vi "TS-60.vi"() -> ()   [LabVIEW 2013]
panel:
  in  "Slide 2":dbl(slide) scale=0.0..10.0
  out "ABC Ind3":bool
  out "ACB Ind 3":bool
  in  "ABC-ACB 3":bool=TRUE
  in  "Slide":dbl(slide) scale=0.0..10.0
  out "ABC Ind 2":bool
  out "ACB Ind 2":bool
  in  "ABC-ACB 2":bool=TRUE
  out "28VDC Ind":bool
  in  "28VDC":bool
  out "SPEED - FPM":dbl format="%3.1f"
  out "DOWNFORCE":dbl format="%1.1f"
  out "TRACTIVE LOAD":dbl format="%1.1f"
  in  "Stop Button":bool
  out "400Hz Ind":bool
  in  "400Hz":bool
  out "ABC Ind":bool
  out "ACB Ind":bool
  in  "ABC-ACB":bool=TRUE
  out "DC AMPS":dbl format="%.3f"
  out "DC VOLTS":dbl format="%-2.1f"
  out "AC FREQUENCY":dbl format="%4.1f"
  out "AC AMPS L3":dbl format="%1.2f"
  out "AC VOLTS L3":dbl format="%3.1f"
  out "AC AMPS L2":dbl format="%1.2f"
  out "AC VOLTS L2":dbl format="%1.1f"
  out "AC AMPS L1":dbl format="%1.2f"
  out "AC VOLTS L1":dbl format="%1.1f"
  in  "DC V":dbl(slide) scale=0.0..30.0
  in  "DC A":dbl(slide) scale=0.0..5.0
  in  "AC FREQ":dbl(slide) scale=0.0..400.0
  in  "AC VOLTS":dbl(slide) scale=0.0..115.0
  in  "AC AMPS":dbl(slide) scale=0.0..25.0
  # "SYSTEM CONTROL"
  # "28VDC"
  # "OFF"
  # "LOAD CONDITION"
  # "DOWNFORCE"
  # "UP"
  # "DOWN"
  # "TRACTION"
  # "ON"
  # "OFF"
  # "400Hz"
  # "OFF"
  # "ABC"
  # "ACB"
  # "POWER CONSUMPTION"
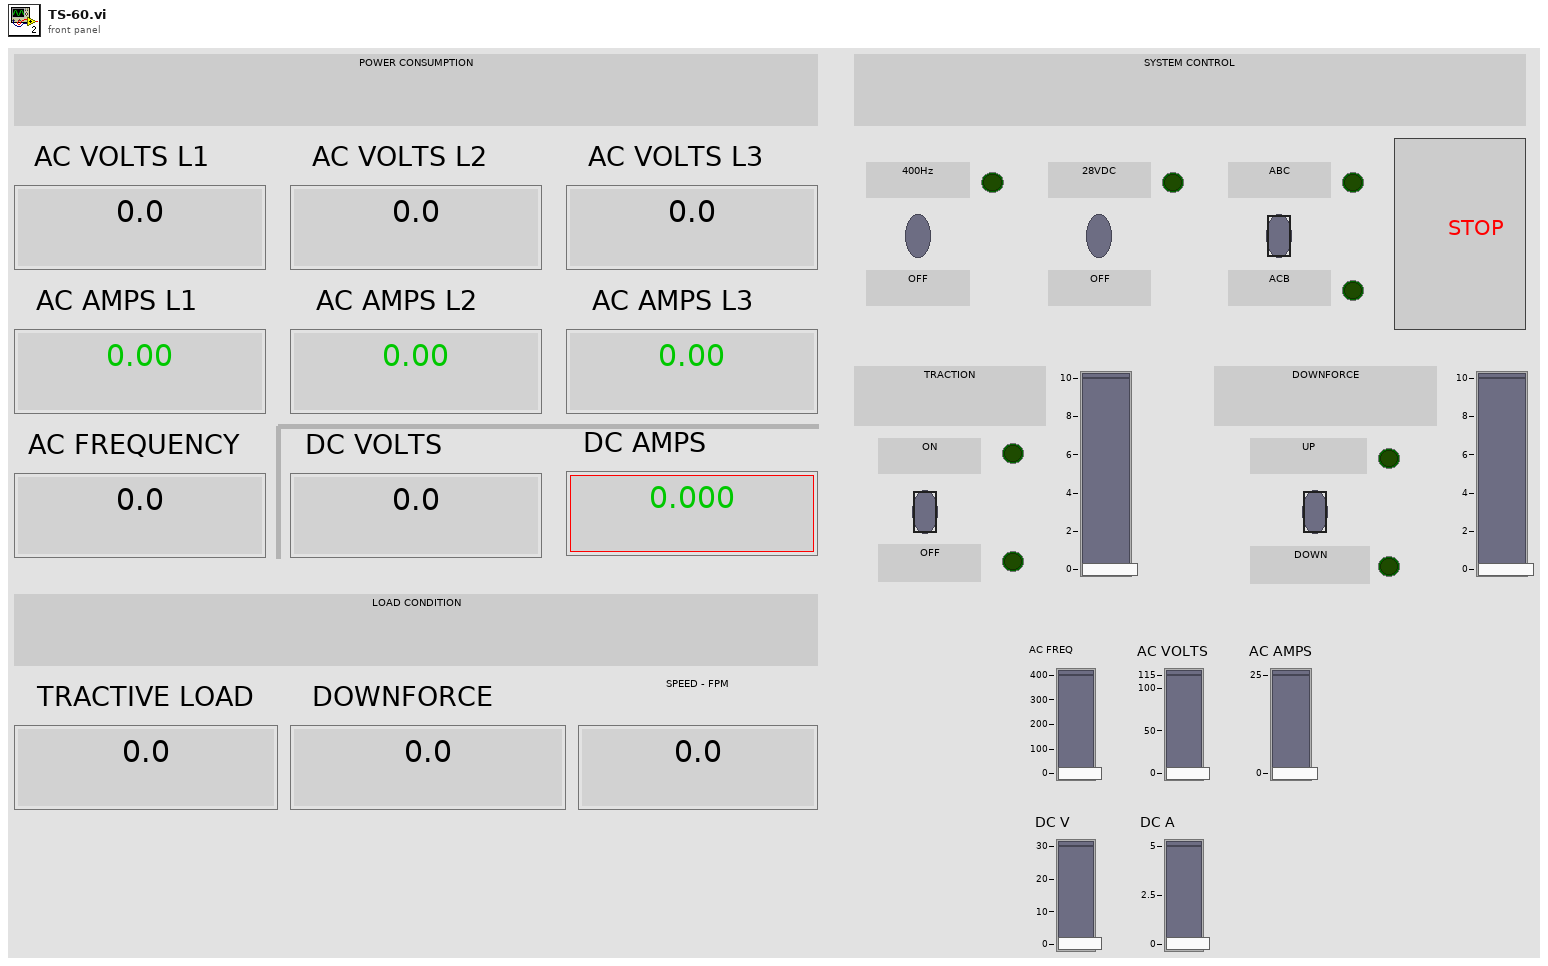
[diagram p1: front panel]
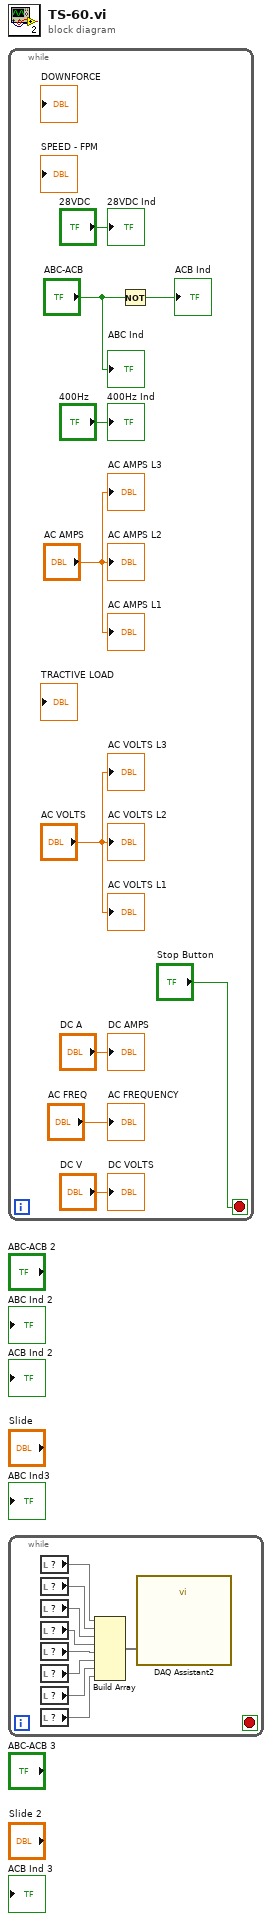
[diagram p0: block diagram]
diagram:
  n1 = while {
    stop <- "Stop Button" stop-if-true
    n2 = Not(x="ABC-ACB") -> (.not. x?=→"ACB Ind":bool)
    "DC VOLTS" <- "DC V"
    "DC AMPS" <- "DC A"
    "AC AMPS L1" <- "AC AMPS"
    "AC VOLTS L1" <- "AC VOLTS"
    "AC VOLTS L2" <- "AC VOLTS"
    "AC AMPS L2" <- "AC AMPS"
    "AC VOLTS L3" <- "AC VOLTS"
    "AC AMPS L3" <- "AC AMPS"
    "AC FREQUENCY" <- "AC FREQ"
    "ABC Ind" <- "ABC-ACB"
    "400Hz Ind" <- "400Hz"
    "28VDC Ind" <- "28VDC"
  }
  n3 = while {
    stop <- _ stop-if-true
    n4 = local read item#-1() -> (w18)
    n5 = local read item#-1() -> (w17)
    n6 = local read item#-1() -> (w16)
    n7 = local read item#-1() -> (w15)
    n8 = local read item#-1() -> (w14)
    n9 = local read item#-1() -> (w13)
    n10 = local read item#-1() -> (w12)
    n11 = local read item#-1() -> (w11)
    n12 = Build Array(w18, w17, w16, w15, w14, w13, w12, w11) -> (w19:void[])
    n13 = call "DAQ Assistant2"("data"=w19) -> ()  [unwired: 17 in, 2 out]
  }
